vi "Static Cleanup.vi"(8 "error in (no error)":errorcluster, 11 "Panel in":refnum<class "Panel.lvclass">) -> (0 "error out":errorcluster)   [LabVIEW 2020, in "OOPanel.lvlib" / "Panel.lvclass"]
uses:
  Panel.lvclass
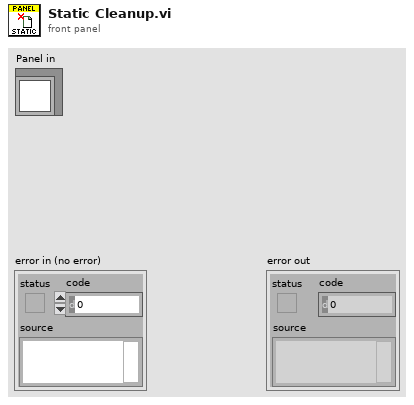
[diagram p1: front panel]
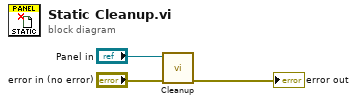
[diagram p0: block diagram]
diagram:
  n1 = call-dynamic "Cleanup.vi"("error in (no error)"="error in (no error)", "Panel in"="Panel in") -> ("error out"=→"error out":errorcluster)  [unwired: 9 in]
